vi "4_4.vi"() -> ()   [LabVIEW 2017]
panel:
  in  "stop":bool
  out "While Loop Iteration":u32
  out "Loop Timing":i32
  in  "Delay":u32
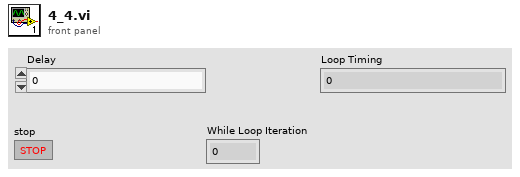
[diagram p1: front panel]
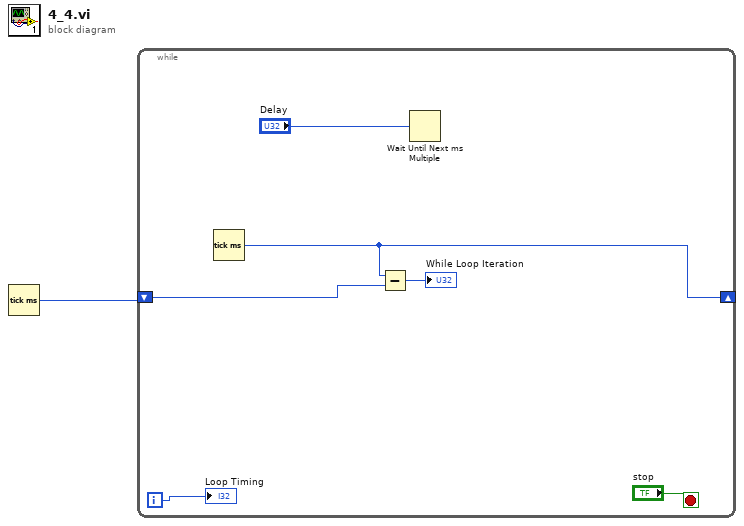
[diagram p0: block diagram]
diagram:
  n1 = Tick Count (ms)() -> (millisecond timer value=w1:u32)
  n2 = while {
    shift-right: [w5] -> _
    shift-left: w1 -> [w6]
    i -> [w2]
    stop <- "stop" stop-if-true
    n3 = Tick Count (ms)() -> (millisecond timer value=w5:u32)
    n4 = Subtract(x=w5, y=w6) -> (x-y=→"While Loop Iteration":u32)
    n5 = Wait Until Next ms Multiple(millisecond multiple="Delay") -> ()  [unwired: 1 out]
    "Loop Timing" <- w2
  }
